vi "qtoPWM.vi"(11 "vq":dbl[](array[numeric])) -> (2 "Numeric 2":dbl, 3 "Numeric":dbl)   [LabVIEW 2024]
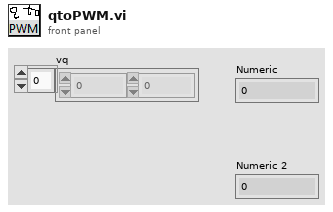
[diagram p1: front panel]
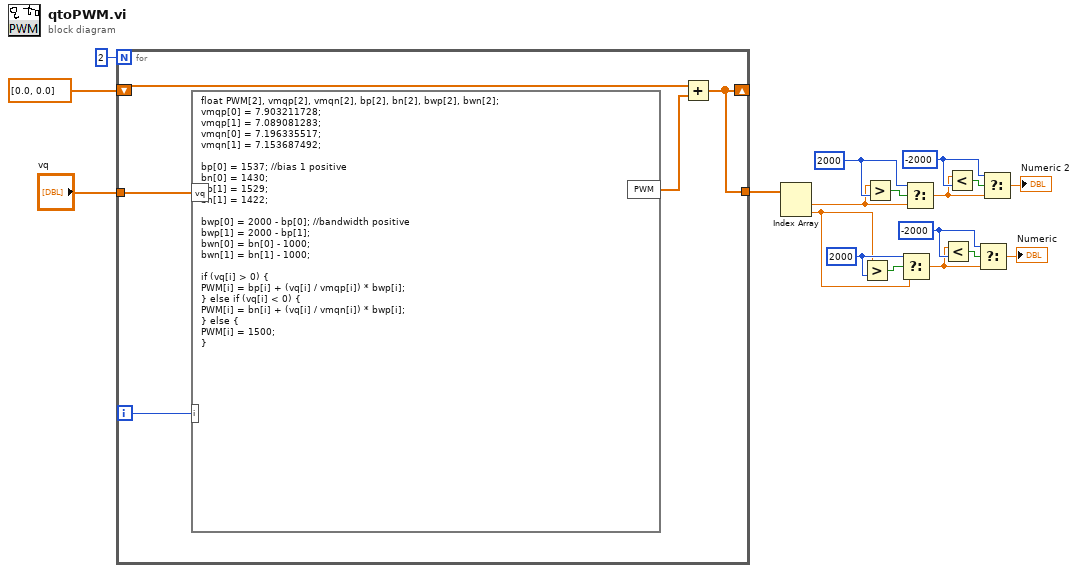
[diagram p0: block diagram]
diagram:
  w4 = -2000
  w6 = 2000
  w10 = -2000
  w13 = 2000
  n1 = for {
    N: 2 -> [_]
    tunnel: "vq" -> [w22]
    tunnel: [w21] -> w16
    shift-right: [w21] -> _
    shift-left: dbl[] [0.0, 0.0] -> [w19]
    i -> [w23]
    n2 = formula code="float PWM[2], vmqp[2], vmqn[2], bp[2], bn[2], bwp[2], bwn[2];\nvmqp[0] = 7.903211728;\nvmqp[1] = 7.089081283;\nvmqn[0] = 7.196335517;\nvmqn[1] = 7.153687492;\n\nbp[0] = 1537; //bias 1 positive\nbn[0] = 1430;\nbp[1] = 1529;\nbn[1] = 1422;\n\nbwp[0] = 2000 - bp[0]; //bandwidth positive\nbwp[1] = 2000 - bp[1];\nbwn[0] = bn[0] - 1000;\nbwn[1] = bn[1] - 1000;\n\nif (vq[i] > 0) {\nPWM[i] = bp[i] + (vq[i] / vmqp[i]) * bwp[i];\n} else if (vq[i] < 0) {\nPWM[i] = bn[i] + (vq[i] / vmqn[i]) * bwp[i];\n} else {\nPWM[i] = 1500;\n}"("vq"=w22, "i"=w23) -> ("PWM"=w20:dbl[])
    n3 = Add(x=w19, y=w20) -> (x+y=w21:dbl[])
  }
  n4 = Index Array(array=w16) -> (element #1=w12:dbl, element #2=w2:dbl)  [unwired: 2 in]
  n5 = Greater?(x=w2, y=w6) -> (0:w7:bool)
  n6 = Greater?(x=w12, y=w13) -> (0:w14:bool)
  n7 = Select(t=w6, s=w7, f=w2) -> (s? t:f=w3:dbl)
  n8 = Select(t=w13, s=w14, f=w12) -> (s? t:f=w9:dbl)
  n9 = Less?(x=w3, y=w4) -> (x < y?=w5:bool)
  n10 = Less?(x=w9, y=w10) -> (x < y?=w11:bool)
  n11 = Select(t=w4, s=w5, f=w3) -> (s? t:f=→"Numeric":dbl)
  n12 = Select(t=w10, s=w11, f=w9) -> (s? t:f=→"Numeric 2":dbl)
